vi "S2C_FPGA_Host2TargetFIFO.vi"   [LabVIEW 2015]
uses:
  <vilib>/rvi/DataTransferAndStorage/Container/XNode/niFpgaContainer.xnode
  <vilib>/rvi/interface/RandomDataEmulation/nirviRandomDataFpgaReadWriteTemplate.vi
  <vilib>/rvi/FIFO/Fifo_Resource/nirvififoEmulationWrite.vi
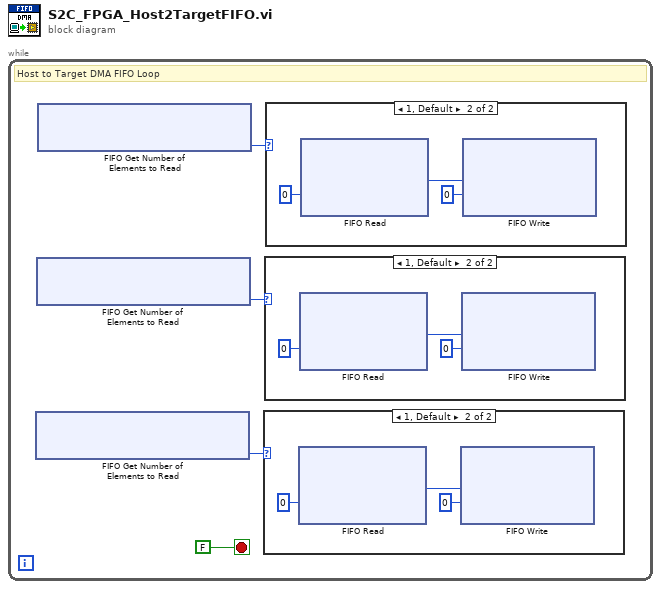
[diagram p0: block diagram]
diagram:
  n1 = while {
    stop <- FALSE stop-if-true
    # "Host to Target DMA FIFO Loop"
    n2 = xnode "FIFO Get Number of Elements to Read"() -> ("Number of Elements to Read"=w1:u32)  [unwired: 1 in, 1 out]
    n3 = xnode "FIFO Get Number of Elements to Read"() -> ("Number of Elements to Read"=w2:u32)  [unwired: 1 in, 1 out]
    n4 = xnode "FIFO Get Number of Elements to Read"() -> ("Number of Elements to Read"=w3:u32)  [unwired: 1 in, 1 out]
    n5 = case shown="1, Default" w1 {
      frame 0 {
      }
      frame 1, Default {
        n6 = xnode "FIFO Read"("Timeout"=0) -> ("Element"=w6:u16)  [unwired: 1 in, 2 out]
        n7 = xnode "FIFO Write"("Element"=w6, "Timeout"=0) -> ()  [unwired: 1 in, 2 out]
      }
    }
    n8 = case shown="1, Default" w2 {
      frame 0 {
      }
      frame 1, Default {
        n9 = xnode "FIFO Read"("Timeout"=0) -> ("Element"=w9:u16)  [unwired: 1 in, 2 out]
        n10 = xnode "FIFO Write"("Element"=w9, "Timeout"=0) -> ()  [unwired: 1 in, 2 out]
      }
    }
    n11 = case shown="1, Default" w3 {
      frame 0 {
      }
      frame 1, Default {
        n12 = xnode "FIFO Read"("Timeout"=0) -> ("Element"=w12:u16)  [unwired: 1 in, 2 out]
        n13 = xnode "FIFO Write"("Element"=w12, "Timeout"=0) -> ()  [unwired: 1 in, 2 out]
      }
    }
  }
